vi "create PlayerUpdaate.vi"(7 "Alive?":bool, 8 "error in (no error)":errorcluster, 10 "Player":refnum<class "Player.lvclass">, 11 "PlayerUpdate in":refnum<class "PlayerUpdate.lvclass">) -> (0 "error out":errorcluster, 3 "PlayerUpdate out":refnum<class "PlayerUpdate.lvclass">)   [LabVIEW 2019, in "PlayerUpdate.lvclass"]
uses:
  PlayerUpdate.lvclass
  Player/Player.lvclass
  PlayerUpdate.lvclass/PlayerUpdate.ctl
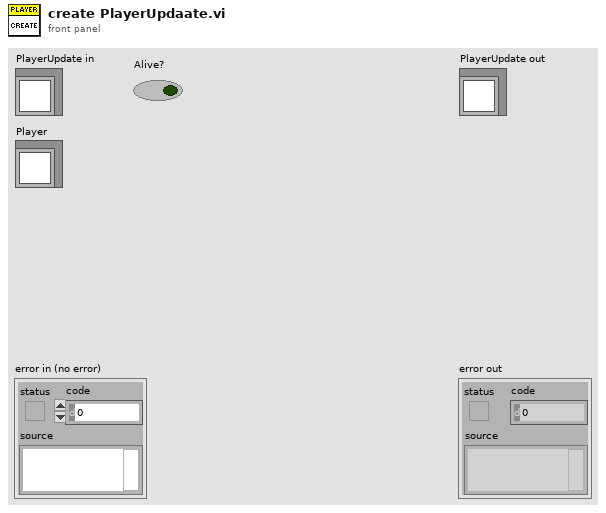
[diagram p1: front panel]
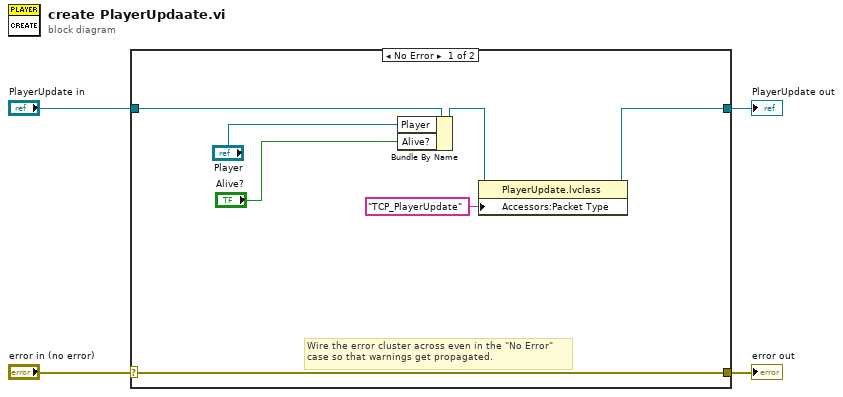
[diagram p0: block diagram]
diagram:
  n1 = case shown="No Error" "error in (no error)" {
    selector: "error in (no error)" -> [w10 w13]
    tunnel: [w10 w13] -> w3
    tunnel: [w6 w12] -> w1
    tunnel: "PlayerUpdate in" -> [w11 w12]
    frame No Error {
      # "Wire the error cluster across even in the \"No Error\"\ncase so that warnings get propagated."
      n2 = Bundle By Name(cluster=w11, "Player"="Player", "Alive?"="Alive?") -> (w7:refnum<class "PlayerUpdate.lvclass">)
      n3 = property class="PlayerUpdate.lvclass"(reference=w7, "Accessors:Packet Type"="TCP_PlayerUpdate" ("Packet Type")) -> (reference out=w6:refnum<class "PlayerUpdate.lvclass">)  [unwired: 1 in, 1 out]
    }
    frame Error {
    }
  }
  "error out" <- w3
  "PlayerUpdate out" <- w1
